vi "Opdracht_1_ZetHexInVolgorde_Hex2Num.vi"(11 "Getallen":string) -> (1 "*(type *) &x":sgl)   [LabVIEW 2018]
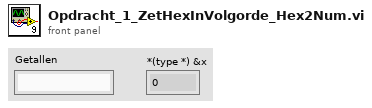
[diagram p1: front panel]
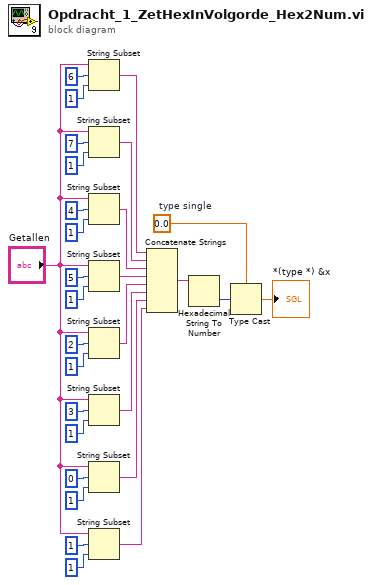
[diagram p0: block diagram]
diagram:
  w12 = sgl 0.0  # type single
  n1 = String Subset(string="Getallen", offset (0)=6, length (rest)=1 ("length (len. of substring)")) -> (substring=w20:string)
  n2 = String Subset(string="Getallen", offset (0)=7, length (rest)=1 ("length (len. of substring)")) -> (substring=w19:string)
  n3 = String Subset(string="Getallen", offset (0)=4, length (rest)=1 ("length (len. of substring)")) -> (substring=w18:string)
  n4 = String Subset(string="Getallen", offset (0)=5, length (rest)=1 ("length (len. of substring)")) -> (substring=w17:string)
  n5 = String Subset(string="Getallen", offset (0)=2 ("length (len. of substring)"), length (rest)=1 ("length (len. of substring)")) -> (substring=w16:string)
  n6 = String Subset(string="Getallen", offset (0)=3, length (rest)=1 ("length (len. of substring)")) -> (substring=w15:string)
  n7 = String Subset(string="Getallen", offset (0)=0, length (rest)=1 ("length (len. of substring)")) -> (substring=w14:string)
  n8 = String Subset(string="Getallen", offset (0)=1, length (rest)=1 ("length (len. of substring)")) -> (substring=w13:string)
  n9 = Concatenate Strings(w20, w19, w18, w17, w16, w15, w14, w13) -> (w2:string)
  n10 = Hexadecimal String To Number(string=w2) -> (number=w3:u32)  [unwired: 2 in, 1 out]
  n11 = Type Cast(type=w12, x=w3) -> (*(type *) &x=→"*(type *) &x":sgl)
